vi "Timer FGV.vi"(9 "Temps cible (s)":dbl, 11 "Commande du timer":T1) -> (1 "Temps écoulé":dbl, 2 "Terminé ?":bool)   [LabVIEW 2009]
doc: "Ce VI est une variable globale fonctionnelle qui garde une trace du temps écoulé depuis qu'une commande Démarrer a été envoyée au VI."
uses:
  TimerCommands.ctl
panel:
  # "Entrée"
  # "Sortie"
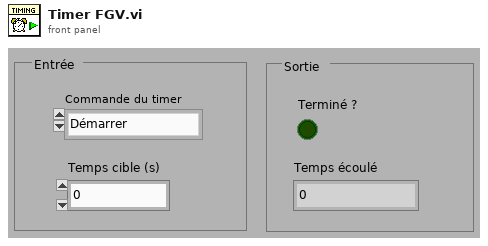
[diagram p1: front panel]
types:
  T1 = typedef "TimerCommands.ctl" = enum16{"Démarrer", "Vérifier le temps"}
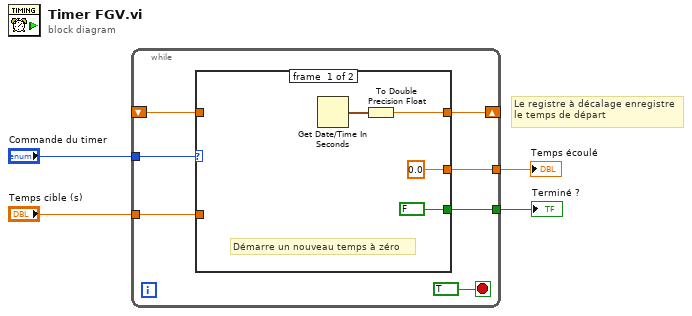
[diagram p0: block diagram]
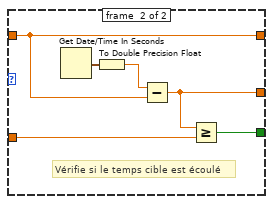
[diagram p2: hidden frame]
diagram:
  # "Le registre à décalage enregistre\nle temps de départ"
  n1 = while "Boucle While" {
    tunnel: "Commande du timer" -> [w11]
    shift-right: [w10] -> _
    shift-left: _ -> [w9]
    tunnel: [w8] -> w3
    tunnel: [w7] -> w2
    tunnel: "Temps cible (s)" -> [w6]
    stop <- TRUE stop-if-true
    n2 = case "Structure Condition" shown="\"Démarrer\", Par défaut" w11 {
      tunnel: [w14 w19] -> w10
      tunnel: w9 -> [_ w19]
      tunnel: [0.0 ("double precision float") w18] -> w8
      tunnel: [FALSE w17] -> w7
      tunnel: w6 -> [_ w16]
      frame #0 {
        # "Démarre un nouveau temps à zéro"
        n3 = Get Date/Time In Seconds() -> (seconds since 1Jan1904=w15:timestamp)
        n4 = To Double Precision Float(number=w15) -> (double precision float=w14:dbl)
      }
      frame #1 {
        # "Vérifie si le temps cible est écoulé"
        n5 = Get Date/Time In Seconds() -> (seconds since 1Jan1904=w21:timestamp)
        n6 = To Double Precision Float(number=w21) -> (double precision float=w20:dbl)
        n7 = Subtract(x=w20, y=w19) -> (x-y=w18:dbl)
        n8 = Greater Or Equal?(x=w18, y=w16) -> (x >= y?=w17:bool)
      }
    }
  }
  "Temps écoulé" <- w3
  "Terminé ?" <- w2
